vi "Set Parent Visible.vi"(8 "error in (no error)":errorcluster, 10 "Parent visible? [T]":bool=TRUE, 11 "IObject in":refnum<class "IObject.lvclass">) -> (0 "error out":errorcluster, 3 "IObject out":refnum<class "IObject.lvclass">)   [LabVIEW 2021, in "IObject.lvclass"]
uses:
  IObject.lvclass
  IObject.lvclass/IObject.ctl
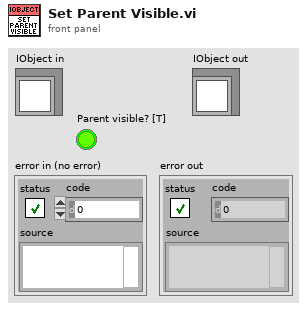
[diagram p1: front panel]
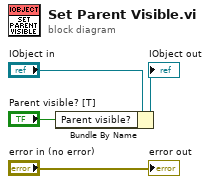
[diagram p0: block diagram]
diagram:
  n1 = Bundle By Name(cluster="IObject in", "Parent visible?"="Parent visible? [T]") -> (→"IObject out":refnum<class "IObject.lvclass">)
  "error out" <- "error in (no error)"
